vi "Asylum_Driver_LithographyObjectPoints.vi"(4 "Abort Notifier":refnum<notifier>, 6 "Interpolation":dbl format="%#_13g", 7 "Writing Setpoint":dbl=0.1 format="%#_13g", 8 "error in (no error)":errorcluster, 9 "Offsets":cluster{"X":dbl, "Y":dbl}, 10 "Pattern Data":T2={"Name"="", "Litho"=[], "Set Resistance"=enum."1G ohm", "Meta"=variant}, 11 "Application":refnum<k7>) -> (0 "error out":errorcluster, 1 "Y":dbl[](array[numeric]), 2 "X":dbl[](array[numeric]), 3 "Application":refnum<k7>)   [LabVIEW 2019]
uses:
  <userlib>/LevyLab/Relay Box/Typedefs/Resistor--enum.ctl
  Asylum_Driver_XYMetersToVoltageArray.vi
  <userlib>/LevyLab/Relay Box/Relay-Box.lvclass
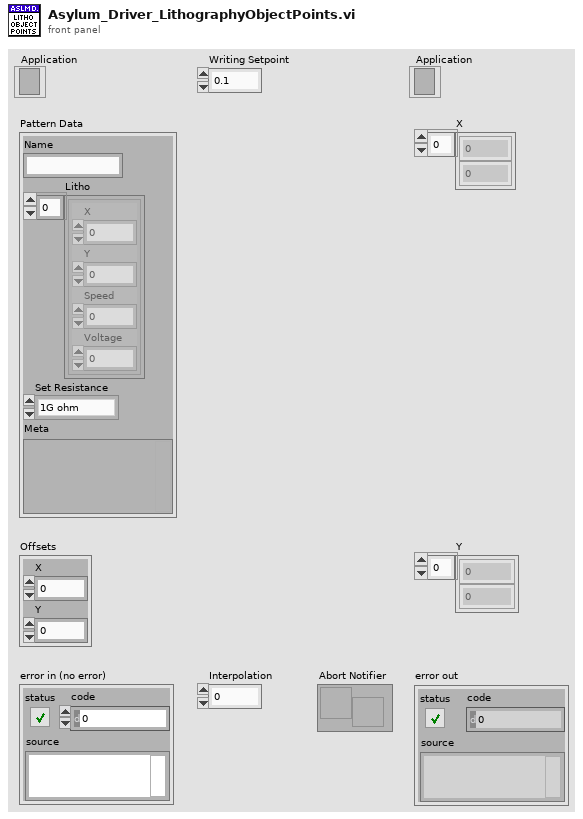
[diagram p1: front panel]
types:
  T1 = typedef "Relay-Box.lvclass/Resistor--enum.ctl" = enum16{"open", "discharge tip", "0 ohms", "100k ohm", "10M ohm", "1G ohm"}
  T2 = cluster{"Name":string, "Litho":cluster{"X":dbl, "Y":dbl, "Speed":dbl, "Voltage":dbl}[], "Set Resistance":T1, "Meta":variant}
  T3 = cluster{"X":dbl, "Y":dbl, "Speed":dbl, "Voltage":dbl}[]
  T4 = cluster{"setpoint":dbl, "pgain":dbl, "igain":dbl, "sgain":dbl}
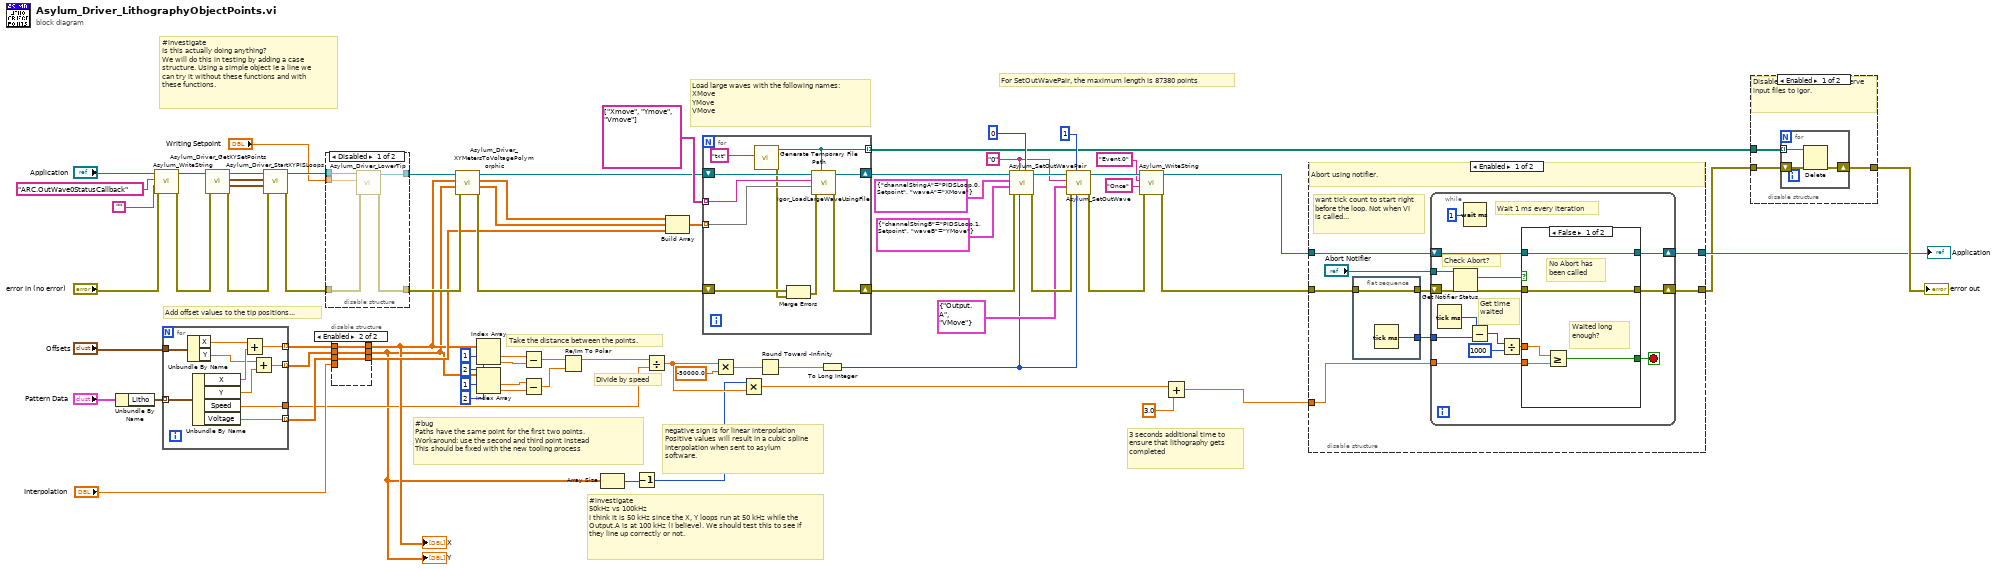
[diagram p0: block diagram]
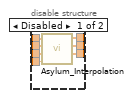
[diagram p2: hidden frame]
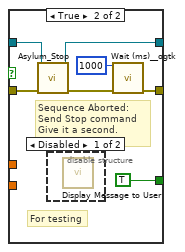
[diagram p5: hidden frame]
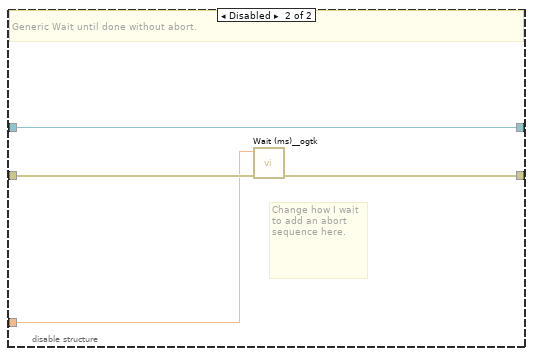
[diagram p7: hidden frame]
diagram:
  w25 = "0" ("eventString")
  # "For SetOutWavePair, the maximum length is 87380 points"
  # "#bug\nPaths have the same point for the first two points. \nWorkaround: use the second and third point instead\nThis should be fixed with the new tooling process"
  # "3 seconds additional time to ensure that lithography gets completed"
  # "Divide by speed"
  # "Load large waves with the following names:\nXMove\nYMove\nVMove"
  # "#investigate\nIs this actually doing anything?\nWe will do this in testing by adding a case structure. Using a simple object ie a line we can try it without these functions and with these functions."
  # "#investigate \n50kHz vs 100kHz\nI think it is 50 kHz since the X, Y loops run at 50 kHz while the Output.A is at 100 kHz (I believe). We should test this to see if they line up correctly or not."
  # "negative sign is for linear interpolation\nPositive values will result in a cubic spline interpolation when sent to asylum software."
  # "Add offset values to the tip positions..."
  # "Take the distance between the points."
  n1 = Unbundle By Name("Pattern Data") -> ("Litho"=w61:T3)
  n2 = call <userlib>:"Asylum_WriteString.vi"("error in (no error)"="error in (no error)", "valueString"="", "parameterName"="ARC.OutWave0StatusCallback", "Application"="Application") -> ("error out"=w72:errorcluster, "Application"=w59:refnum<k7>)  [unwired: 6 in]
  n3 = for {
    tunnel: w61 -> [w83] mode=indexing
    tunnel: [w82] -> w10
    tunnel: [w81] -> w28 mode=indexing
    tunnel: "Offsets" -> [w79]
    tunnel: [w75] -> w54 mode=indexing
    tunnel: [w74] -> w49 mode=indexing
    n4 = Unbundle By Name(w79) -> ("X"=w77:dbl, "Y"=w76:dbl)
    n5 = Unbundle By Name(w83) -> ("X"=w80:dbl, "Y"=w78:dbl, "Speed"=w82:dbl, "Voltage"=w81:dbl)
    n6 = Add(x=w77, y=w80) -> (x+y=w75:dbl)
    n7 = Add(x=w76, y=w78) -> (x+y=w74:dbl)
  }
  n8 = call "Asylum_Driver_GetXYSetPoints.vi"("error in (no error)"=w72, "Application"=w59) -> ("error out"=w73:errorcluster, "Y PIS Controls"=w22:T4, "X PIS Controls"=w23:T4, "Application"=w21:refnum<k7>)  [unwired: 6 in]
  n9 = call "Asylum_Driver_StartXYPISLoops.vi"("error in (no error)"=w73, "Y PIS Controls"=w22, "X PIS Controls"=w23, "Application"=w21) -> ("error out"=w65:errorcluster, "Application"=w20:refnum<k7>)  [unwired: 6 in]
  n10 = disable-structure shown="Disabled" {
    disable-tunnel: [w84 w89] -> w69
    disable-tunnel: w65 -> [w85 w89]
    disable-tunnel: [w88 w90] -> w52
    disable-tunnel: w20 -> [w87 w90]
    disable-tunnel: "Writing Setpoint" -> [w86 _]
    frame Disabled {
      n11 = call "Asylum_Driver_LowerTip.vi"("error in (no error)"=w85, "Z Setpoint"=w86, "Application"=w87) -> ("error out"=w84:errorcluster, "Application"=w88:refnum<k7>)  [unwired: 7 in]
    }
    frame Enabled {
      # "Put the tip down in initialize lithography object"
    }
  }
  n12 = disable-structure shown="Enabled" {
    disable-tunnel: w54 -> [w97 w100]
    disable-tunnel: w49 -> [w96 w99]
    disable-tunnel: "Interpolation" -> [w95 _]
    disable-tunnel: w28 -> [w94 w98]
    disable-tunnel: [w93 w98] -> w27
    disable-tunnel: [w92 w100] -> w16
    disable-tunnel: [w91 w99] -> w5
    frame Disabled {
      n13 = call "Asylum_Interpolation.vi"("X"=w97, "Y"=w96, "V"=w94, "Interpolation"=w95) -> ("X"=w92:dbl[], "Y"=w91:dbl[], "V"=w93:dbl[])  [unwired: 4 in]
    }
    frame Enabled {
    }
  }
  "Y" <- w5
  "X" <- w16
  n14 = call-poly "Asylum_Driver_XYMetersToVoltagePolymorphic.vi"("error in (no error)"=w69, "Y Coordinate"=w5, "X Coordinate"=w16, "Application"=w52) -> ("error out"=w66:errorcluster, "Y Voltage"=w50:dbl[], "X Voltage"=w1:dbl[], "Application"=w51:refnum<k7>)  [unwired: 4 in]
  n15 = Index Array(array=w16, index #1=1 ("index"), index #2=2 ("index")) -> (element #1=w47:dbl, element #2=w46:dbl)
  n16 = Index Array(array=w5, index #1=1 ("index"), index #2=2 ("index")) -> (element #1=w45:dbl, element #2=w44:dbl)
  n17 = Subtract(x=w47, y=w46) -> (x-y=w43:dbl)
  n18 = Subtract(x=w45, y=w44) -> (x-y=w42:dbl)
  n19 = Re/Im To Polar(2:w42, 3:w43) -> (1:w41:dbl)  [unwired: 1 out]
  n20 = Array Size(array=w5) -> (size(s)=w11:i32)
  n21 = Decrement(x=w11) -> (x-1=w9:i32)
  n22 = Divide(x=w41, y=w10) -> (x/y=w29:dbl)
  n23 = Build Array(w1, w50, w27) -> (w55:dbl[][])
  n24 = for {
    tunnel: w55 -> [w108] mode=indexing
    shift-right: [w110] -> w70
    shift-left: w66 -> [w103]
    tunnel: string[] ["Xmove", "Ymove", "Vmove"] -> [w107] mode=indexing
    shift-right: [w106] -> w38
    shift-left: w51 -> [w109]
    tunnel: [w104] -> w24 mode=indexing
    n25 = call <vilib>:"Generate Temporary File Path.vi"("Temporary File Extension (tmp)"="txt") -> ("error out"=w102:errorcluster, "Unique Temporary File Path"=w104:path)  [unwired: 9 in]
    n26 = Merge Errors(w103, w102) -> (w101:errorcluster)
    n27 = call <userlib>:"Igor_LoadLargeWaveUsingFile.vi"("Path"=w104, "error in"=w101, "Wave"=w108, "Wavename"=w107, "Application"=w109) -> ("error out"=w110:errorcluster, "Application"=w106:refnum<k7>)  [unwired: 5 in]
  }
  n28 = Multiply(x=w29, y=-50000.0) -> (x*y=w3:dbl)
  n29 = Multiply(x=w9, y=w29) -> (x*y=w8:dbl)
  n30 = Round Toward -Infinity(1:w3) -> (0:w2:dbl)
  n31 = To Long Integer(number=w2) -> (32bit integer=w26:i32)
  n32 = call <userlib>:"Asylum_SetOutWavePair.vi"("whichBank"=0, "interpolation"=w26, "eventString"=w25, "error in (no error)"=w70, "Wave B"=cluster{"channelStringB":string, "waveB":string} {"channelStringB"="PIDSLoop.1.Setpoint", "waveB"="YMove"}, "Wave A"=cluster{"channelStringA":string, "waveA":string} {"channelStringA"="PIDSLoop.0.Setpoint", "waveA"="XMove"}, "Application"=w38) -> ("error out"=w68:errorcluster, "Application"=w34:refnum<k7>)  [unwired: 3 in]
  n33 = call <userlib>:"Asylum_SetOutWave.vi"("interpolation"=w26, "whichBank"=1, "error in (no error)"=w68, "Wave"=cluster{"channelString":string, "wave":string} {"channelString"="Output.A", "wave"="VMove"}, "eventString"=w25, "Application"=w34) -> ("error out"=w67:errorcluster, "Application"=w32:refnum<k7>)  [unwired: 4 in]
  n34 = call <userlib>:"Asylum_WriteString.vi"("error in (no error)"=w67, "valueString"="Once", "parameterName"="Event.0", "Application"=w32) -> ("error out"=w64:errorcluster, "Application"=w18:refnum<k7>)  [unwired: 6 in]
  n35 = Add(x=w8, y=3.0) -> (x+y=w7:dbl)
  n36 = disable-structure shown="Enabled" {
    disable-tunnel: w64 -> [w117 w151]
    disable-tunnel: w7 -> [w111 w148]
    disable-tunnel: w18 -> [w113 w149]
    disable-tunnel: [w112 w149] -> w19
    disable-tunnel: [w116 w150] -> w17
    frame Enabled {
      # "want tick count to start right before the loop. Not when VI is called..."
      # "Abort using notifier."
      n37 = flat-sequence {
        tunnel: [w119] -> w114
        tunnel: w117 -> [w120]
        tunnel: [w120] -> w118
        frame #0 {
          n38 = Tick Count (ms)() -> (millisecond timer value=w119:u32)
        }
      }
      n39 = while {
        tunnel: "Abort Notifier" -> [w132]
        shift-right: [w129] -> w112
        shift-left: w113 -> [w130]
        shift-right: [w134] -> w116
        shift-left: w118 -> [w133]
        tunnel: w114 -> [w126]
        tunnel: w111 -> [w124]
        stop <- w128 stop-if-true
        # "Check Abort?"
        # "Wait 1 ms every iteration"
        # "Get time waited"
        n40 = Tick Count (ms)() -> (millisecond timer value=w127:u32)
        n41 = Get Notifier Status(notifier=w132, error in (no error)=w133) -> (current notification=w131:bool, error out=w135:errorcluster)  [unwired: 3 out]
        n42 = Wait (ms)(milliseconds to wait=u32 1) -> ()  [unwired: 1 out]
        n43 = Subtract(x=w127, y=w126) -> (x-y=w123:u32)
        n44 = Divide(x=w123, y=u32 1000) -> (x/y=w121:dbl)
        n45 = case shown="False" w131 {
          tunnel: w130 -> [w139 w146]
          tunnel: [w139 w145] -> w129
          tunnel: w135 -> [w140 w147]
          tunnel: [w140 w142] -> w134
          tunnel: [w137 TRUE] -> w128
          tunnel: w124 -> [w138 _]
          tunnel: w121 -> [w136 _]
          frame False {
            # "No Abort has been called"
            # "Waited long enough?"
            n46 = Greater Or Equal?(x=w136, y=w138) -> (x >= y?=w137:bool)
          }
          frame True {
            # "For testing"
            # "Sequence Aborted:\nSend Stop command\nGive it a second."
            n47 = call <userlib>:"Asylum_Stop.vi"("error in (no error)"=w147, "Application"=w146) -> ("error out"=w143:errorcluster, "Application"=w145:refnum<k7>)  [unwired: 8 in]
            n48 = disable-structure shown="Disabled" {
              frame Disabled {
                n49 = call "Display Message to User"() -> ()  [unwired: 10 in, 2 out]
              }
              frame Enabled {
              }
            }
            n50 = call <userlib>:"Wait (ms)__ogtk.vi"("error in (no error)"=w143, "milliseconds to wait"=u32 1000) -> ("error out"=w142:errorcluster)  [unwired: 8 in, 1 out]
          }
        }
      }
    }
    frame Disabled {
      # "Change how I wait to add an abort sequence here."
      # "Generic Wait until done without abort."
      n51 = call <userlib>:"Wait (ms)__ogtk.vi"("error in (no error)"=w151, "milliseconds to wait"=w148) -> ("error out"=w150:errorcluster)  [unwired: 8 in, 1 out]
    }
  }
  "Application" <- w19
  n52 = disable-structure shown="Enabled" {
    disable-tunnel: [w154 w158] -> w63
    disable-tunnel: w24 -> [w153 _]
    disable-tunnel: w17 -> [w152 w158]
    frame Enabled {
      # "Disable this diagram to preserve input files to igor."
      n53 = for {
        tunnel: w153 -> [w155] mode=indexing
        shift-right: [w156] -> w154
        shift-left: w152 -> [w157]
        n54 = Delete(path (use dialog)=w155, error in=w157) -> (error out=w156:errorcluster)  [unwired: 3 in, 2 out]
      }
    }
    frame Disabled {
    }
  }
  "error out" <- w63
